vi "NI VeriStand - Remove Item Property.vi"(8 "error in (no error)":errorcluster, 10 "Property Name":string, 11 "Item Ref in":T1 format="%.0x") -> (0 "error out":errorcluster, 1 "Removed":bool, 3 "Item Ref out":T1 format="%.0x")   [LabVIEW 2020, in "Custom Device API.lvlib"]
doc: "Removes the property specified by <B>Property Name</B> from a custom device item."
uses:
  <vilib>/NI VeriStand/Custom Device API/Custom Device API.lvlib
  <vilib>/NI VeriStand/Custom Device API/Custom Device Item Ref.ctl
  22a1df45-0b90-4f75-bbff-dafc71b17d27.vi
  <vilib>/NI VeriStand/Custom Device API/Custom Device Offline Path.vi
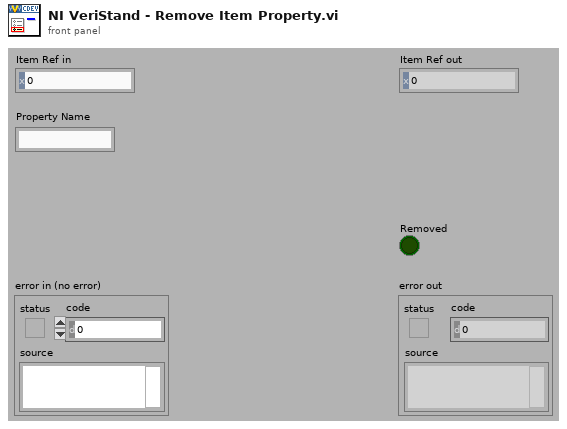
[diagram p1: front panel]
types:
  T1 = typedef "Custom Device API.lvlib/Custom Device Item Ref.ctl" = u64
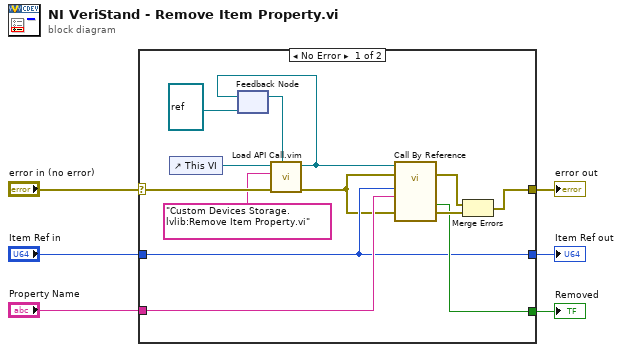
[diagram p0: block diagram]
diagram:
  n1 = case shown="No Error" "error in (no error)" {
    selector: "error in (no error)" -> [w12 w21]
    tunnel: [w18 w21] -> w6
    tunnel: "Item Ref in" -> [w15 w20]
    tunnel: "Property Name" -> [w17 _]
    tunnel: [w15 w20] -> w3
    tunnel: [w16 _] -> w2
    frame No Error {
      n2 = control-ref of="This VI"() -> (w13:refnum<vi>)
      n3 = feedback #1(refnum<vi> refnum ("type specifier VI Refnum (for type only)")) -> (w14:refnum<vi>)
      n4 = call "Load API Call.vim"("VI reference in"=w14, "error in (no error)"=w12, "VI qualified name"="Custom Devices Storage.lvlib:Remove Item Property.vi", "Caller VI ref"=w13) -> ("error out"=w11:errorcluster, "VI reference"=w10:refnum<vi>)  [unwired: 6 in]
      n5 = feedback-in #1(w10) -> ()
      n6 = call-by-ref "?"(reference=w10, error in=w11, 8:"error in (no error)"=w11, "Property Name"=w17, "Item Ref in"=w15) -> (error out=w7:errorcluster, 0:"error out"=w19:errorcluster, "Removed"=w16:bool)  [unwired: 6 in, 2 out]
      n7 = Merge Errors(w7, w19) -> (w18:errorcluster)
    }
    frame Error {
    }
  }
  "Item Ref out" <- w3
  "error out" <- w6
  "Removed" <- w2
